vi "PQfastSelectCommand.vi"(8 "error in (no error)":errorcluster, 10 "SelectString":string, 11 "conn":u32) -> (0 "database_status_message":T1, 1 "data":string[][](array[string]), 2 "column_names":string[](array[string]), 3 "conn_out":u32, 4 "error out":errorcluster)   [LabVIEW 2019]
uses:
  libpqutility.lvlib
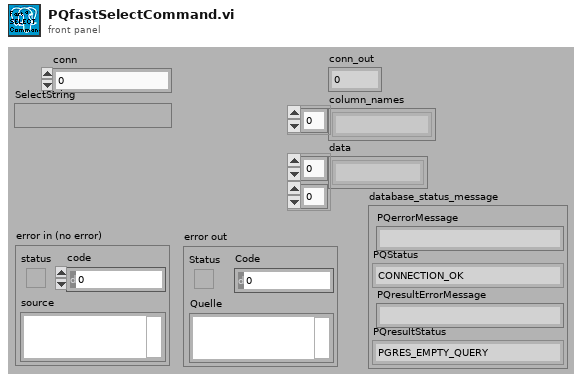
[diagram p1: front panel]
types:
  T1 = cluster{"PQerrorMessage":string, "PQStatus":enum16{"CONNECTION_OK", "CONNECTION_BAD", "CONNECTION_STARTED", "CONNECTION_MADE", "CONNECTION_AWAITING_RESPONSE", "CONNECTION_AUTH_OK", "CONNECTION_SETENV", "CONNECTION_SSL_STARTUP", "CONNECTION_NEEDED"}, "PQresultErrorMessage":string, "PQresultStatus":enum16{"PGRES_EMPTY_QUERY", "PGRES_COMMAND_OK", "PGRES_TUPLES_OK", "PGRES_COPY_OUT", "PGRES_COPY_IN", "PGRES_BAD_RESPONSE", "PGRES_NONFATAL_ERROR", "PGRES_FATAL_ERROR"}}
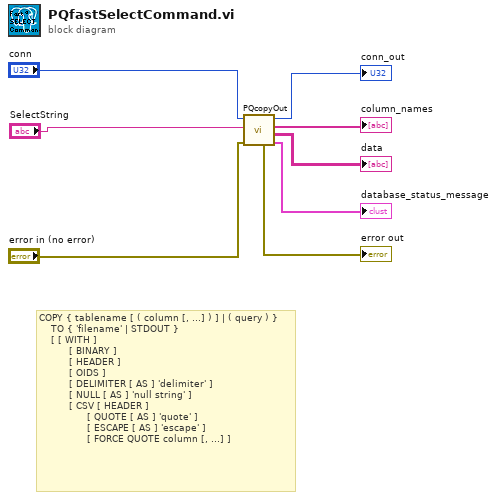
[diagram p0: block diagram]
diagram:
  # "COPY { tablename [ ( column [, ...] ) ] | ( query ) }\n    TO { 'filename' | STDOUT }\n    [ [ WITH ] \n          [ BINARY ]\n          [ HEADER ]\n          [ OIDS ]\n          [ DELIMITER [ AS ] 'delimiter' ]\n          [ NULL [ AS ] 'null string' ]\n          [ CSV [ HEADER ]\n                [ QUOTE [ AS ] 'quote' ] \n                [ ESCAPE [ AS ] 'escape' ]\n                [ FORCE QUOTE column [, ...] ]"
  n1 = call "PQcopyOut.vi"("error in (no error)"="error in (no error)", "query"="SelectString", "conn"="conn") -> ("database_status_message"=→"database_status_message":T1, "data"=→"data":string[][], "column_names"=→"column_names":string[], "conn_out"=→"conn_out":u32, "error out"=→"error out":errorcluster)  [unwired: 4 in]
